vi "Unzip.vi"(8 "error in":errorcluster, 10 "Path":path, 11 "Archivist in":refnum<class "Archivist.lvclass">) -> (0 "error out":errorcluster, 3 "Archivist out":refnum<class "Archivist.lvclass">)   [LabVIEW 2019, in "Archivist.lvclass"]
uses:
  Archivist.lvclass
  <userlib>/_OpenG.lib/lvzip/lvzip.llb/subVI/ZLIB Extract All Files To Dir (Path)__ogtk.vi
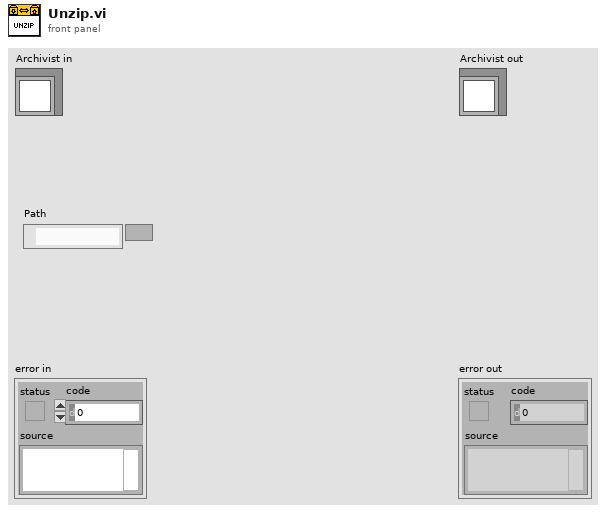
[diagram p1: front panel]
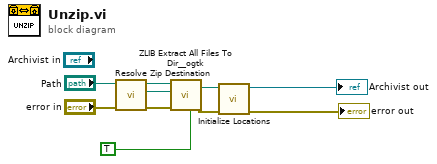
[diagram p0: block diagram]
diagram:
  n1 = call "Resolve Zip Destination.vi"("error in (no error)"="error in", "Zip File In"="Path") -> ("error out"=w5:errorcluster, "Destination"=w3:path, "Zip File Out"=w4:path)  [unwired: 7 in]
  n2 = call-poly <userlib>:"ZLIB Extract All Files To Dir__ogtk.vi"("overwrite (F)"=TRUE, "error in (no error)"=w5, "destination directory (archive name without ending)"=w3, "archive name (file dialog)"=w4) -> ("error out"=w6:errorcluster, "destination directory out"=w10:path)  [unwired: 5 in, 1 out]
  n3 = call "Initialize Locations.vi"("error in"=w6, "Save Location"=w10) -> ("error out"=→"error out":errorcluster, "Archivist out"=→"Archivist out":refnum<class "Archivist.lvclass">)  [unwired: 8 in]
